vi "averagePos.vi"(7 "robotPos":cluster{"xPos":dbl, "yPos":dbl, "Theta":dbl}={"xPos"=278.12308270038665, "yPos"=314.23015698912945, "Theta"=-158.01372232471553}, 10 "readPositions":T1(array[cluster])) -> (2 "newRobotPos":cluster{"xPos":dbl, "yPos":dbl, "Theta":dbl})   [LabVIEW 2016]
panel:
  out "a +/- b":cluster{"xPos":dbl, "yPos":dbl, "Theta":dbl}={"xPos"=nan, "yPos"=nan, "Theta"=nan}
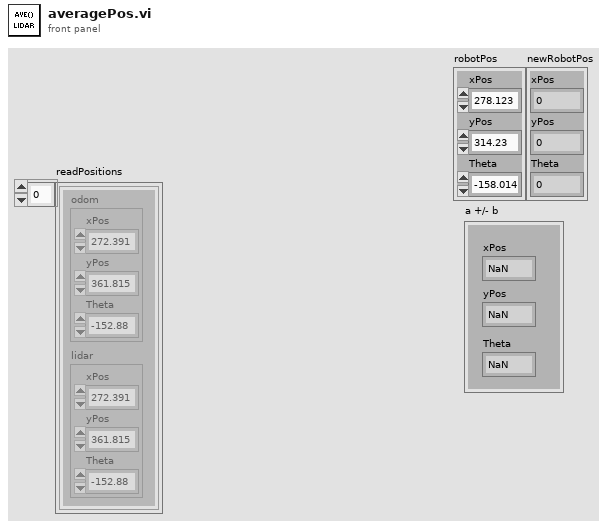
[diagram p1: front panel]
types:
  T1 = cluster{"odom":cluster{"xPos":dbl, "yPos":dbl, "Theta":dbl}, "lidar":cluster{"xPos":dbl, "yPos":dbl, "Theta":dbl}}[]
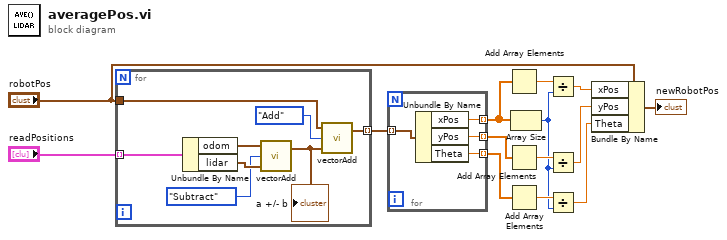
[diagram p0: block diagram]
diagram:
  n1 = for {
    tunnel: "readPositions" -> [w22] mode=indexing
    tunnel: "robotPos" -> [w17]
    tunnel: [w16] -> w13 mode=indexing
    n2 = Unbundle By Name(w22) -> ("odom"=w21:cluster{"xPos":dbl, "yPos":dbl, "Theta":dbl}, "lidar"=w20:cluster{"xPos":dbl, "yPos":dbl, "Theta":dbl})
    n3 = call "vectorAdd.vi"("b"=w20, "operation"=enum16{"Subtract", "Add"}."Subtract", "a"=w21) -> ("a +/- b"=w18:cluster{"xPos":dbl, "yPos":dbl, "Theta":dbl})  [unwired: 1 in]
    "a +/- b" <- w18
    n4 = call "vectorAdd.vi"("b"=w18, "operation"=enum16{"Subtract", "Add"}."Add", "a"=w17) -> ("a +/- b"=w16:cluster{"xPos":dbl, "yPos":dbl, "Theta":dbl})  [unwired: 1 in]
  }
  n5 = for {
    tunnel: w13 -> [w26] mode=indexing
    tunnel: [w25] -> w2 mode=indexing
    tunnel: [w24] -> w10 mode=indexing
    tunnel: [w23] -> w5 mode=indexing
    n6 = Unbundle By Name(w26) -> ("xPos"=w25:dbl, "yPos"=w24:dbl, "Theta"=w23:dbl)
  }
  n7 = Add Array Elements(numeric array=w2) -> (sum=w12:dbl)
  n8 = Add Array Elements(numeric array=w10) -> (sum=w11:dbl)
  n9 = Add Array Elements(numeric array=w5) -> (sum=w4:dbl)
  n10 = Array Size(array=w2) -> (size(s)=w3:i32)
  n11 = Divide(x=w12, y=w3) -> (x/y=w8:dbl)
  n12 = Divide(x=w11, y=w3) -> (x/y=w7:dbl)
  n13 = Divide(x=w4, y=w3) -> (x/y=w1:dbl)
  n14 = Bundle By Name(cluster="robotPos", "xPos"=w8, "yPos"=w7, "Theta"=w1) -> (→"newRobotPos":cluster{"xPos":dbl, "yPos":dbl, "Theta":dbl})
